vi "CAN Uninitialize.vi"(8 "错误输入（无错误）":errorcluster, 11 "Channel":u16) -> (0 "错误输出":errorcluster, 2 "Channel 2":u16, 3 "function return":u32)   [LabVIEW 2021, in "PCANBasic.lvlib"]
doc: "TPCANStatus __stdcall CAN_Uninitialize(\n TPCANHandle Channel);"
uses:
  PCANBasic.lvlib
  <userlib>/PCANBasic/PCANBasic.dll
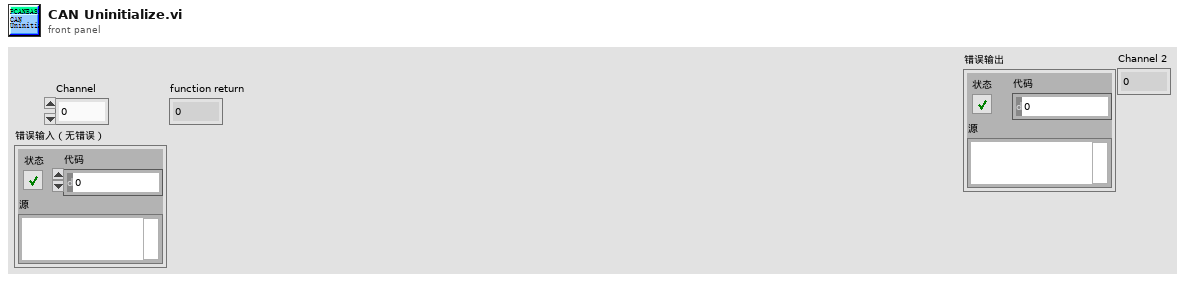
[diagram p1: front panel]
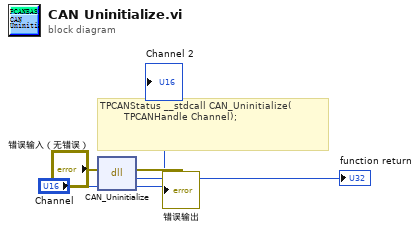
[diagram p0: block diagram]
diagram:
  # "TPCANStatus __stdcall CAN_Uninitialize(\n        TPCANHandle Channel);"
  n1 = dll-call lib="C:/Program Files (x86)/National Instruments/LabVIEW 2021/user.lib/PCANBasic/PCANBasic.*" fn="CAN_Uninitialize"(error in="错误输入（无错误）", "Channel"="Channel") -> (error out=→"错误输出":errorcluster, →"function return":u32, "Channel"=→"Channel 2":u16)  [unwired: 2 in, 1 out]
